vi "DAQmx.Enumerate Chassis.vi"(8 "error in (no error)":errorcluster) -> (0 "error out":errorcluster, 3 "Chassis and Controllers":T1[](array[typedef]))   [LabVIEW 2019, in "DAQmx.lvclass"]
uses:
  DAQmx.lvclass
  typedefs/DeviceInfo--Cluster.ctl
  <vilib>/nisyscfg/Filter Mode.ctl
  <vilib>/nisyscfg/Close (Filter).vi
  <vilib>/nisyscfg/Close (Hardware).vi
  <vilib>/nisyscfg/Close (System).vi
  <resource>/objmgr/nicontrollersysapi.rc
  <vilib>/nisyscfg/nisyscfg.lvlib
  <resource>/objmgr/nisysapi.rc
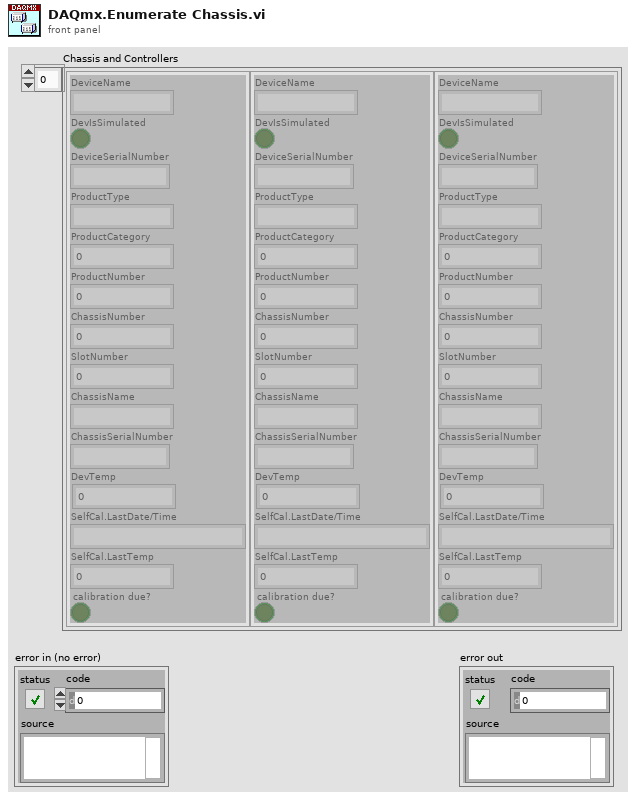
[diagram p1: front panel]
types:
  T1 = typedef "DAQmx.lvclass/DeviceInfo--Cluster.ctl" = cluster{"DeviceName":string, "DevIsSimulated":bool, "DeviceSerialNumber":string, "ProductType":string, "ProductCategory":i32, "ProductNumber":u32, "ChassisNumber":u32, "SlotNumber":u32, "ChassisName":string, "ChassisSerialNumber":string, "DevTemp":dbl, "SelfCal.LastDate/Time":string, "SelfCal.LastTemp":dbl, "calibration due?":bool}
  T2 = typedef "nisyscfg.lvlib/Filter Mode.ctl" = i32
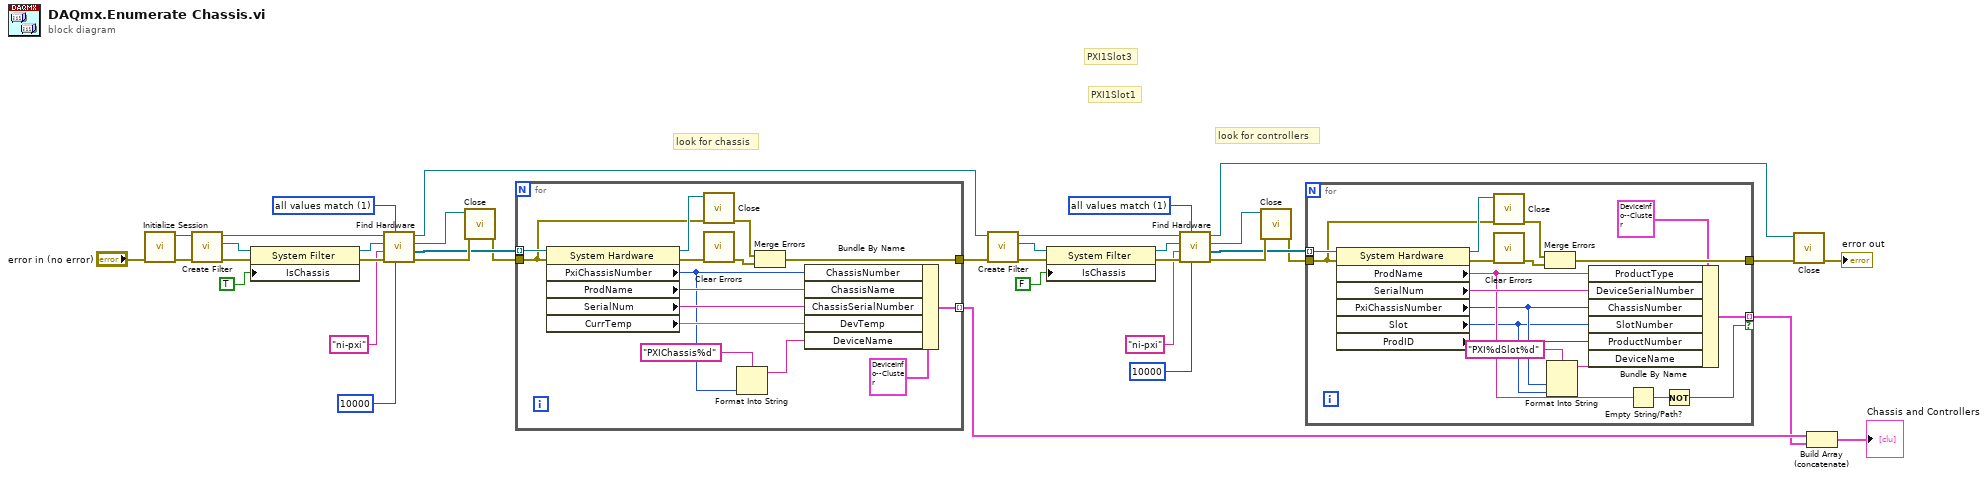
[diagram p0: block diagram]
diagram:
  w20 = T2 1 items=["all values match"=1, "any value matches"=2, "values do not match"=3, "all properties exist"=4] ("Filter Mode (all values match)")
  w28 = T2 1 items=["all values match"=1, "any value matches"=2, "values do not match"=3, "all properties exist"=4] ("Filter Mode (all values match)")
  # "look for chassis"
  # "look for controllers"
  # "PXI1Slot1"
  # "PXI1Slot3"
  n1 = call <vilib>:"Initialize Session.vi"("error in (no error)"="error in (no error)") -> ("error out"=w25:errorcluster, "Session out"=w27:refnum<k21>)  [unwired: 9 in]
  n2 = call <vilib>:"Create Filter.vi"("error in (no error)"=w25, "Session in"=w27) -> ("error out"=w36:errorcluster, "Filter out"=w35:refnum<k20>, "Session out"=w34:refnum<k21>)  [unwired: 7 in]
  n3 = property class="System Filter"(reference=w35, error in=w36, "IsChassis"=TRUE ("Is Chassis")) -> (reference out=w33:refnum<k20>, error out=w32:errorcluster)
  n4 = call <vilib>:"Find Hardware.vi"("Remote Timeout (300,000 ms)"=u32 10000, "Filter Mode (all values match)"=w28, "error in (no error)"=w32, "Experts"="ni-pxi", "Filter in"=w33, "Session in"=w34) -> ("error out"=w23:errorcluster, "Resources out"=w9:refnum<k20>[], "Filter out"=w24:refnum<k20>, "Session out"=w6:refnum<k21>)  [unwired: 2 in]
  n5 = call-poly <vilib>:"Close.vi"("error in (no error)"=w23, "Filter in"=w24) -> ("error out"=w8:errorcluster)  [unwired: 9 in]
  n6 = for {
    tunnel: w9 -> [w52] mode=indexing
    tunnel: w8 -> [w47]
    tunnel: [w50] -> w7
    tunnel: [w43] -> w5 mode=indexing
    n7 = property class="System Hardware"(reference=w52, error in=w47) -> (reference out=w51:refnum<k20>, error out=w49:errorcluster, "PxiChassisNumber"=w40:u32, "ProdName"=w45:string, "SerialNum"=w42:string, "CurrTemp"=w41:dbl)
    n8 = call-poly <vilib>:"Close.vi"("error in (no error)"=w47, "Resource in"=w51) -> ("error out"=w48:errorcluster)  [unwired: 9 in]
    n9 = call <vilib>:"Clear Errors.vi"("error in (no error)"=w49) -> ("error out"=w46:errorcluster)  [unwired: 5 in, 1 out]
    n10 = Format Into String(format string="PXIChassis%d" ("DeviceName"), w40) -> (resulting string=w38:string)  [unwired: 2 in, 1 out]
    n11 = Merge Errors(w48, w46) -> (w50:errorcluster)
    n12 = Bundle By Name(cluster=T1 {"DeviceName"="", "DevIsSimulated"=FALSE, "DeviceSerialNumber"="", "ProductType"="", "ProductCategory"=0, "ProductNumber"=0, "ChassisNumber"=0, "SlotNumber"=0, "ChassisName"="", "ChassisSerialNumber"="", "DevTemp"=0.0, "SelfCal.LastDate/Time"="", "SelfCal.LastTemp"=0.0, "calibration due?"=FALSE} ("Device"), "ChassisNumber"=w40, "ChassisName"=w45, "ChassisSerialNumber"=w42, "DevTemp"=w41, "DeviceName"=w38) -> (w43:T1)
  }
  n13 = call <vilib>:"Create Filter.vi"("error in (no error)"=w7, "Session in"=w6) -> ("error out"=w14:errorcluster, "Filter out"=w15:refnum<k20>, "Session out"=w16:refnum<k21>)  [unwired: 7 in]
  n14 = property class="System Filter"(reference=w15, error in=w14, "IsChassis"=FALSE ("Is Chassis")) -> (reference out=w17:refnum<k20>, error out=w18:errorcluster)
  n15 = call <vilib>:"Find Hardware.vi"("Remote Timeout (300,000 ms)"=u32 10000, "Filter Mode (all values match)"=w20, "error in (no error)"=w18, "Experts"="ni-pxi", "Filter in"=w17, "Session in"=w16) -> ("error out"=w22:errorcluster, "Resources out"=w12:refnum<k20>[], "Filter out"=w21:refnum<k20>, "Session out"=w1:refnum<k21>)  [unwired: 2 in]
  n16 = call-poly <vilib>:"Close.vi"("error in (no error)"=w22, "Filter in"=w21) -> ("error out"=w11:errorcluster)  [unwired: 9 in]
  n17 = for {
    tunnel: w12 -> [w70] mode=indexing
    tunnel: w11 -> [w65]
    tunnel: [w68] -> w2
    tunnel: [w61] -> w4 mode=indexing if=w58
    n18 = property class="System Hardware"(reference=w70, error in=w65) -> (reference out=w69:refnum<k20>, error out=w67:errorcluster, "ProdName"=w60:string, "SerialNum"=w62:string, "PxiChassisNumber"=w55:u32, "Slot"=w54:i32, "ProdID"=w57:u32)
    n19 = call-poly <vilib>:"Close.vi"("error in (no error)"=w65, "Resource in"=w69) -> ("error out"=w66:errorcluster)  [unwired: 9 in]
    n20 = call <vilib>:"Clear Errors.vi"("error in (no error)"=w67) -> ("error out"=w64:errorcluster)  [unwired: 5 in, 1 out]
    n21 = Merge Errors(w66, w64) -> (w68:errorcluster)
    n22 = Format Into String(format string="PXI%dSlot%d" ("DeviceName"), w55, w54) -> (resulting string=w53:string)  [unwired: 2 in, 1 out]
    n23 = Bundle By Name(cluster=T1 {"DeviceName"="", "DevIsSimulated"=FALSE, "DeviceSerialNumber"="", "ProductType"="", "ProductCategory"=0, "ProductNumber"=0, "ChassisNumber"=0, "SlotNumber"=0, "ChassisName"="", "ChassisSerialNumber"="", "DevTemp"=0.0, "SelfCal.LastDate/Time"="", "SelfCal.LastTemp"=0.0, "calibration due?"=FALSE} ("Device"), "ProductType"=w60, "DeviceSerialNumber"=w62, "ChassisNumber"=w55, "SlotNumber"=w54, "ProductNumber"=w57, "DeviceName"=w53) -> (w61:T1)
    n24 = Empty String/Path?(string/path=w60) -> (empty?=w59:bool)
    n25 = Not(x=w59) -> (.not. x?=w58:bool)
  }
  n26 = call-poly <vilib>:"Close.vi"("error in (no error)"=w2, "Session in"=w1) -> ("error out"=→"error out":errorcluster)  [unwired: 9 in]
  n27 = Build Array (concatenate)(w5, w4) -> (→"Chassis and Controllers":T1[])
